vi "grid position.vi"   [LabVIEW 2022 SP3]
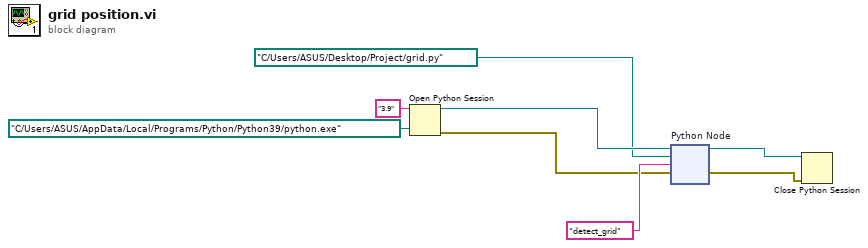
[diagram p0: block diagram]
diagram:
  n1 = Open Python Session(python version="3.9" ("Python version"), python path=path "C:/Users/ASUS/AppData/Local/Programs/Python/Python39/python.exe" ("Python path")) -> (session out=w3:refnum<k35>, error out=w2:errorcluster)  [unwired: 1 in]
  n2 = node "Python Node"(w3, path "C:/Users/ASUS/Desktop/Project/grid.py" ("module path"), "detect_grid" ("function name"), w2) -> (w6:refnum<k35>, w5:errorcluster)  [unwired: 2 in, 2 out]
  n3 = Close Python Session(session in=w6, error in=w5) -> ()  [unwired: 1 out]
